vi "Commit Transaction.vi"(8 "error in":errorcluster, 11 "DB-SQLite in":refnum<class "DB-SQLite.lvclass">) -> (0 "error out":errorcluster, 3 "DB-SQLite out":refnum<class "DB-SQLite.lvclass">)   [LabVIEW 2020, in "hse-db-sqlite.lvlib" / "DB-SQLite.lvclass"]
doc: "____\nHAMPEL SOFTWARE ENGINEERING v1.4.0 (2023-12-19 09:52)"
uses:
  DB-SQLite.lvclass
  DB-SQLite.lvclass/DB-SQLite.ctl
  <vilib>/drjdpowell/SQLite Library/Transaction Helpers/Transaction.lvlib
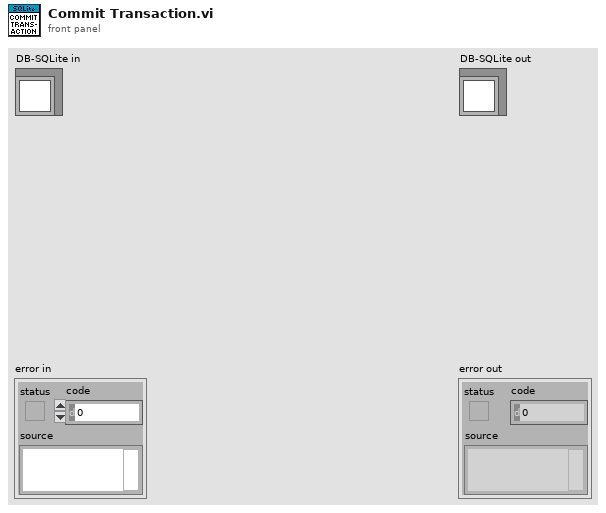
[diagram p1: front panel]
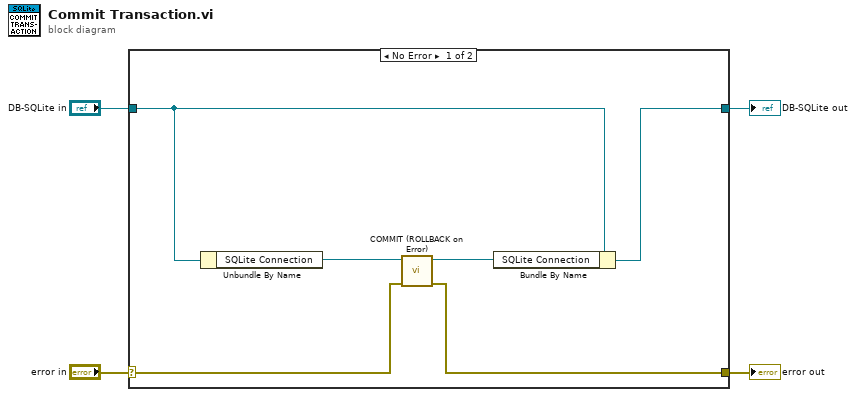
[diagram p0: block diagram]
diagram:
  n1 = case shown="No Error" "error in" {
    selector: "error in" -> [w10 w12]
    tunnel: [w9 w12] -> w3
    tunnel: [w6 w11] -> w1
    tunnel: "DB-SQLite in" -> [w7 w11]
    frame No Error {
      n2 = Unbundle By Name(w7) -> ("SQLite Connection"=w8:refnum<class "Connection.lvclass">)
      n3 = call <vilib>:"COMMIT (ROLLBACK on Error).vi"("error in (no error)"=w10, "SQLite Connection in"=w8) -> ("error out"=w9:errorcluster, "SQLite Connection"=w5:refnum<class "Connection.lvclass">)  [unwired: 8 in]
      n4 = Bundle By Name(cluster=w7, "SQLite Connection"=w5) -> (w6:refnum<class "DB-SQLite.lvclass">)
    }
    frame Error {
    }
  }
  "error out" <- w3
  "DB-SQLite out" <- w1
